vi "Q Image Blocks (SubVI).vi"(7 "Image Size":T1={"Height"=512, "Width"=512} {"Width" step=8; "Height" step=8}, 11 "Data to Disk":T2) -> (3 "Image Blocks":u8[](array[numeric]))   [LabVIEW 2015]
uses:
  Controls (HOST)/Data to Disk Bundle.ctl
  Controls (HOST)/Image Size.ctl
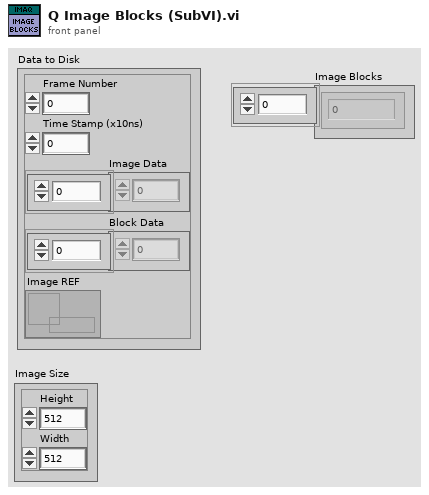
[diagram p1: front panel]
types:
  T1 = typedef "Image Size.ctl" = cluster{"Height":u16, "Width":u16}
  T2 = typedef "Data to Disk Bundle.ctl" = cluster{"Frame Number":u64, "Time Stamp (x10ns)":u64, "Image Data":u64[], "Block Data":u64[], "Image REF":refnum<data-value>}
  T3 = enum16{"big-endian, network order", "native, host order", "little-endian"}
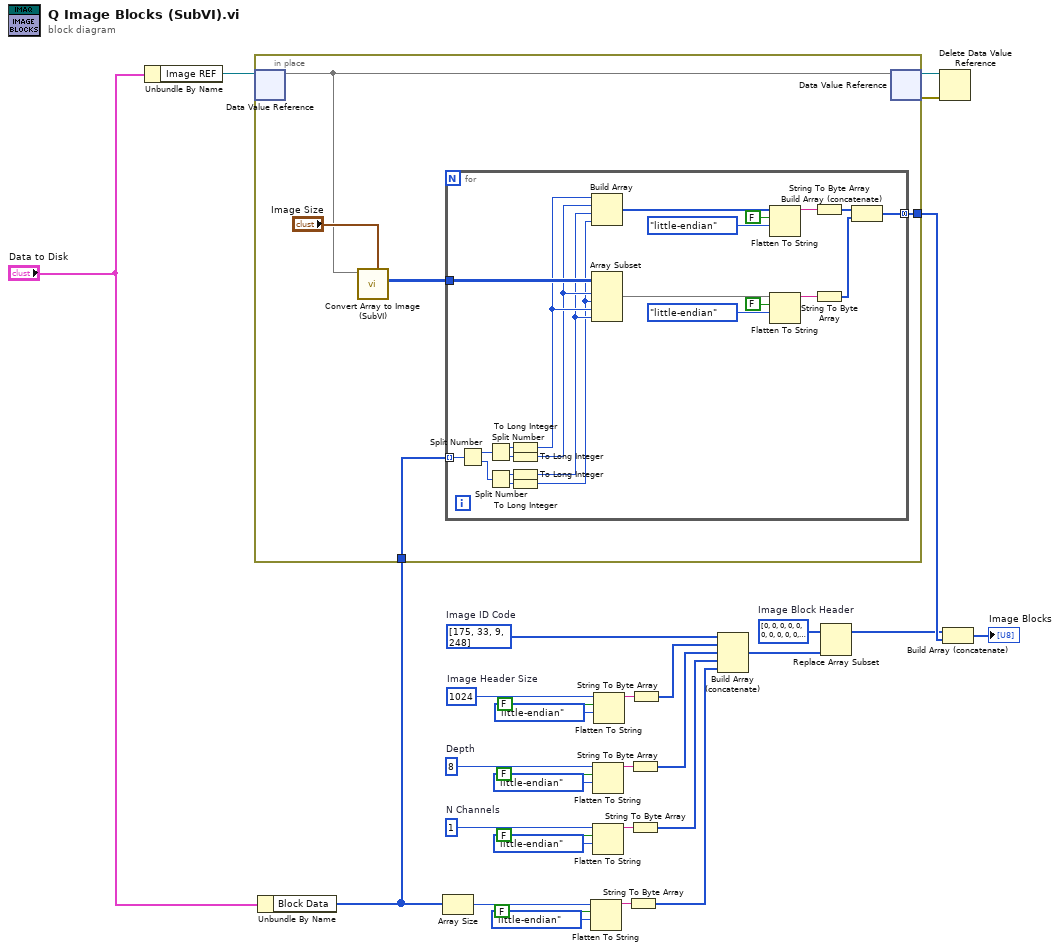
[diagram p0: block diagram]
diagram:
  w20 = 1  # N Channels
  w21 = 8  # Depth
  w30 = 1024  # Image Header Size
  w31 = u8[] [0, 0, 0, 0, 0, 0, 0, 0, 0, 0, 0, 0, 0, 0, 0, 0, 0, 0, 0, 0, 0, 0, 0, 0, 0, 0, 0, 0, 0, 0, 0, 0, 0, 0, 0, 0, 0, 0, 0, 0, 0, 0, 0, 0, 0, 0, 0, 0, 0, 0, 0, 0, 0, 0, 0, 0, 0, 0, 0, 0, 0, 0, 0, 0, 0, 0, 0, 0, 0, 0, 0, 0, 0, 0, 0, 0, 0, 0, 0, 0, 0, 0, 0, 0, 0, 0, 0, 0, 0, 0, 0, 0, 0, 0, 0, 0, 0, 0, 0, 0, 0, 0, 0, 0, 0, 0, 0, 0, 0, 0, 0, 0, 0, 0, 0, 0, 0, 0, 0, 0, 0, 0, 0, 0, 0, 0, 0, 0, 0, 0, 0, 0, 0, 0, 0, 0, 0, 0, 0, 0, 0, 0, 0, 0, 0, 0, 0, 0, 0, 0, 0, 0, 0, 0, 0, 0, 0, 0, 0, 0, 0, 0, 0, 0, 0, 0, 0, 0, 0, 0, 0, 0, 0, 0, 0, 0, 0, 0, 0, 0, 0, 0, 0, 0, 0, 0, 0, 0, 0, 0, 0, 0, 0, 0, 0, 0, 0, 0, 0, 0, 0, 0, 0, 0, 0, 0, 0, 0, 0, 0, 0, 0, 0, 0, 0, 0, 0, 0, 0, 0, 0, 0, 0, 0, 0, 0, 0, 0, 0, 0, 0, 0, 0, 0, 0, 0, 0, 0, 0, 0, 0, 0, 0, 0, 0, 0, 0, 0, 0, 0, 0, 0, 0, 0, 0, 0, 0, 0, 0, 0, 0, 0, 0, 0, 0, 0, 0, 0, 0, 0, 0, 0, 0, 0, 0, 0, 0, 0, 0, 0, 0, 0, 0, 0, 0, 0, 0, 0, 0, 0, 0, 0, 0, 0, 0, 0, 0, 0, 0, 0, 0, 0, 0, 0, 0, 0, 0, 0, 0, 0, 0, 0, 0, 0, 0, 0, 0, 0, 0, 0, 0, 0, 0, 0, 0, 0, 0, 0, 0, 0, 0, 0, 0, 0, 0, 0, 0, 0, 0, 0, 0, 0, 0, 0, 0, 0, 0, 0, 0, 0, 0, 0, 0, 0, 0, 0, 0, 0, 0, 0, 0, 0, 0, 0, 0, 0, 0, 0, 0, 0, 0, 0, 0, 0, 0, 0, 0, 0, 0, 0, 0, 0, 0, 0, 0, 0, 0, 0, 0, 0, 0, 0, 0, 0, 0, 0, 0, 0, 0, 0, 0, 0, 0, 0, 0, 0, 0, 0, 0, 0, 0, 0, 0, 0, 0, 0, 0, 0, 0, 0, 0, 0, 0, 0, 0, 0, 0, 0, 0, 0, 0, 0, 0, 0, 0, 0, 0, 0, 0, 0, 0, 0, 0, 0, 0, 0, 0, 0, 0, 0, 0, 0, 0, 0, 0, 0, 0, 0, 0, 0, 0, 0, 0, 0, 0, 0, 0, 0, 0, 0, 0, 0, 0, 0, 0, 0, 0, 0, 0, 0, 0, 0, 0, 0, 0, 0, 0, 0, 0, 0, 0, 0, 0, 0, 0, 0, 0, 0, 0, 0, 0, 0, 0, 0, 0, 0, 0, 0, 0, 0, 0, 0, 0, 0, 0, 0, 0, 0, 0, 0, 0, 0, 0, 0, 0, 0, 0, 0, 0, 0, 0, 0, 0, 0, 0, 0, 0, 0, 0, 0, 0, 0, 0, 0, 0, 0, 0, 0, 0, 0, 0, 0, 0, 0, 0, 0, 0, 0, 0, 0, 0, 0, 0, 0, 0, 0, 0, 0, 0, 0, 0, 0, 0, 0, 0, 0, 0, 0, 0, 0, 0, 0, 0, 0, 0, 0, 0, 0, 0, 0, 0, 0, 0, 0, 0, 0, 0, 0, 0, 0, 0, 0, 0, 0, 0, 0, 0, 0, 0, 0, 0, 0, 0, 0, 0, 0, 0, 0, 0, 0, 0, 0, 0, 0, 0, 0, 0, 0, 0, 0, 0, 0, 0, 0, 0, 0, 0, 0, 0, 0, 0, 0, 0, 0, 0, 0, 0, 0, 0, 0, 0, 0, 0, 0, 0, 0, 0, 0, 0, 0, 0, 0, 0, 0, 0, 0, 0, 0, 0, 0, 0, 0, 0, 0, 0, 0, 0, 0, 0, 0, 0, 0, 0, 0, 0, 0, 0, 0, 0, 0, 0, 0, 0, 0, 0, 0, 0, 0, 0, 0, 0, 0, 0, 0, 0, 0, 0, 0, 0, 0, 0, 0, 0, 0, 0, 0, 0, 0, 0, 0, 0, 0, 0, 0, 0, 0, 0, 0, 0, 0, 0, 0, 0, 0, 0, 0, 0, 0, 0, 0, 0, 0, 0, 0, 0, 0, 0, 0, 0, 0, 0, 0, 0, 0, 0, 0, 0, 0, 0, 0, 0, 0, 0, 0, 0, 0, 0, 0, 0, 0, 0, 0, 0, 0, 0, 0, 0, 0, 0, 0, 0, 0, 0, 0, 0, 0, 0, 0, 0, 0, 0, 0, 0, 0, 0, 0, 0, 0, 0, 0, 0, 0, 0, 0, 0, 0, 0, 0, 0, 0, 0, 0, 0, 0, 0, 0, 0, 0, 0, 0, 0, 0, 0, 0, 0, 0, 0, 0, 0, 0, 0, 0, 0, 0, 0, 0, 0, 0, 0, 0, 0, 0, 0, 0, 0, 0, 0, 0, 0, 0, 0, 0, 0, 0, 0, 0, 0, 0, 0, 0, 0, 0, 0, 0, 0, 0, 0, 0, 0, 0, 0, 0, 0, 0, 0, 0, 0, 0, 0, 0, 0, 0, 0, 0, 0, 0, 0, 0, 0, 0, 0, 0, 0, 0, 0, 0, 0, 0, 0, 0, 0, 0, 0, 0, 0, 0, 0, 0, 0, 0, 0, 0, 0, 0, 0, 0, 0, 0, 0, 0, 0, 0, 0, 0, 0, 0, 0, 0, 0, 0, 0, 0, 0, 0, 0, 0, 0, 0, 0, 0, 0, 0, 0, 0, 0, 0, 0, 0, 0, 0, 0, 0, 0, 0, 0, 0, 0, 0, 0, 0, 0, 0, 0, 0, 0, 0, 0, 0, 0, 0, 0, 0, 0, 0, 0, 0, 0, 0, 0, 0, 0, 0, 0, 0, 0, 0, 0, 0, 0, 0, 0, 0, 0, 0, 0, 0, 0, 0, 0, 0, 0, 0, 0, 0, 0, 0, 0, 0, 0, 0, 0, 0, 0, 0, 0, 0, 0, 0, 0, 0, 0, 0, 0, 0]  # Image Block Header
  w26 = u8[] [175, 33, 9, 248]  # Image ID Code
  n1 = Unbundle By Name("Data to Disk") -> ("Image REF"=w3:refnum<data-value>)
  n2 = Unbundle By Name("Data to Disk") -> ("Block Data"=w5:u64[])
  n3 = in-place {
    in-place-border: [w36] -> w9
    in-place-border: w5 -> [w35]
    n4 = in-place-dvr #1(w3) -> (w32:u64[])  [unwired: 1 out]
    n5 = call "Convert Array to Image (SubVI).vi"("Image Size"="Image Size", "Image Array In"=w32) -> ("Image Array Out"=w34:u8[][])  [unwired: 9 in]
    n6 = for {
      tunnel: w35 -> [w59] mode=indexing
      tunnel: w34 -> [w56]
      tunnel: [w47] -> w36 mode=concatenating
      n7 = Split Number(x=w59) -> (hi(x)=w57:u32, lo(x)=w58:u32)
      n8 = Split Number(x=w57) -> (hi(x)=w46:u16, lo(x)=w53:u16)
      n9 = Split Number(x=w58) -> (hi(x)=w55:u16, lo(x)=w54:u16)
      n10 = To Long Integer(number=w46) -> (32bit integer=w45:i32)
      n11 = To Long Integer(number=w53) -> (32bit integer=w44:i32)
      n12 = To Long Integer(number=w55) -> (32bit integer=w43:i32)
      n13 = To Long Integer(number=w54) -> (32bit integer=w42:i32)
      n14 = Build Array(w45, w44, w43, w42) -> (w50:i32[])
      n15 = Array Subset(array=w56, index (row)=w44, length (row)=w42, index (col)=w45, length (col)=w43) -> (w38:u8[][])
      n16 = Flatten To String(anything=w50, prepend array or string size? (T)=FALSE, byte order (0:big-endian, network order)=T3."little-endian") -> (data string=w52:string)  [unwired: 1 in, 2 out]
      n17 = Flatten To String(anything=w38, prepend array or string size? (T)=FALSE, byte order (0:big-endian, network order)=T3."little-endian") -> (data string=w39:string)  [unwired: 1 in, 2 out]
      n18 = String To Byte Array(string=w52) -> (unsigned byte array=w51:u8[])
      n19 = String To Byte Array(string=w39) -> (unsigned byte array=w37:u8[])
      n20 = Build Array (concatenate)(w51, w37) -> (w47:u8[])
    }
    n21 = in-place-dvr #1(w32) -> (w1:refnum<data-value>, w2:errorcluster)
  }
  n22 = Array Size(array=w5) -> (size(s)=w6:i32)
  n23 = Flatten To String(anything=w6, prepend array or string size? (T)=FALSE, byte order (0:big-endian, network order)=T3."little-endian") -> (data string=w16:string)  [unwired: 1 in, 2 out]
  n24 = Flatten To String(anything=w21, prepend array or string size? (T)=FALSE, byte order (0:big-endian, network order)=T3."little-endian") -> (data string=w24:string)  [unwired: 1 in, 2 out]
  n25 = Flatten To String(anything=w20, prepend array or string size? (T)=FALSE, byte order (0:big-endian, network order)=T3."little-endian") -> (data string=w17:string)  [unwired: 1 in, 2 out]
  n26 = Flatten To String(anything=w30, prepend array or string size? (T)=FALSE, byte order (0:big-endian, network order)=T3."little-endian") -> (data string=w27:string)  [unwired: 1 in, 2 out]
  n27 = String To Byte Array(string=w16) -> (unsigned byte array=w11:u8[])
  n28 = String To Byte Array(string=w24) -> (unsigned byte array=w13:u8[])
  n29 = String To Byte Array(string=w17) -> (unsigned byte array=w12:u8[])
  n30 = String To Byte Array(string=w27) -> (unsigned byte array=w25:u8[])
  n31 = Build Array (concatenate)(w26, w25, w13, w12, w11) -> (w10:u8[])
  n32 = Replace Array Subset(array=w31, new element=w10) -> (w7:u8[])  [unwired: 1 in]
  n33 = Delete Data Value Reference(data value reference=w1, error in=w2) -> ()  [unwired: 2 out]
  n34 = Build Array (concatenate)(w7, w9) -> (→"Image Blocks":u8[])
